vi "List Buckets.vi"() -> ()   [LabVIEW 2015]
doc: "Demonstrates how to list all of the Amazon S3 buckets you own."
uses:
  Typedefs/AMZ_S3_AWS Credentials.ctl
  LV Interface for Amazon S3.lvlib
panel:
  in  "Secret Key":string
  in  "Access Key":string
  out "Buckets":i32(listbox)
  # "Overview: Demonstrates how to list all Amazon S3 buckets created by an authenticated user.\nRequirements: LabVIEW Interface for Amazon S3 toolkit and a registered Amazon AWS account\nInstructions:\n1. Specify the Access Key and Secret Key for your AWS account. You can create an account at http://aws.amazon.com.\n2. Run the VI. All the buckets associated with your account should be listed in the Buckets indicator."
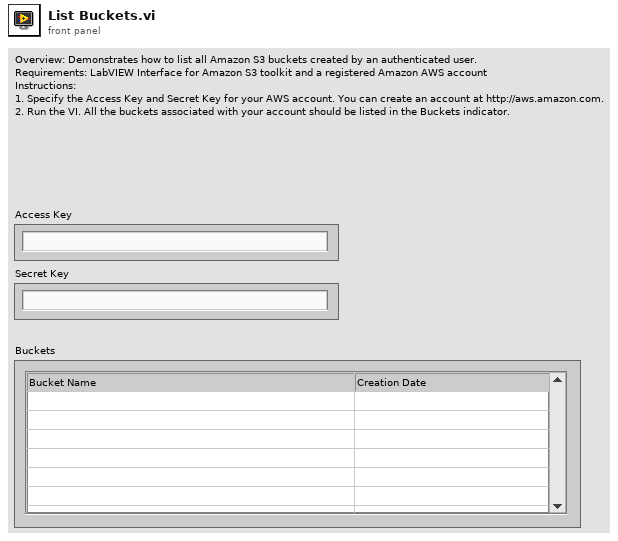
[diagram p1: front panel]
types:
  T1 = typedef "LV Interface for Amazon S3.lvlib/AMZ_S3_AWS Credentials.ctl" = cluster{"Access Key":string, "Secret Key":string}
  T2 = typedef "LV Interface for Amazon S3.lvlib/AMZ_S3_API_Bucket.ctl" = cluster{"Name":string, "CreationDate":timestamp}
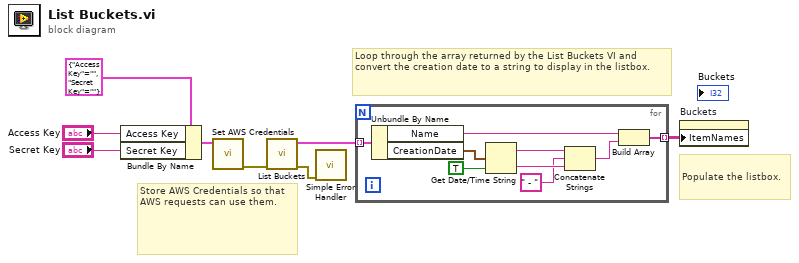
[diagram p0: block diagram]
diagram:
  # "Populate the listbox."
  # "Loop through the array returned by the List Buckets VI and convert the creation date to a string to display in the listbox."
  # "Store AWS Credentials so that AWS requests can use them."
  n1 = Bundle By Name(cluster=T1 {"Access Key"="", "Secret Key"=""} ("AWS Credentials in"), "Access Key"="Access Key", "Secret Key"="Secret Key") -> (w2:T1)
  n2 = call "Set AWS Credentials.vi"("AWS Credentials in"=w2) -> ("error out"=w8:errorcluster)  [unwired: 10 in]
  n3 = call "List Buckets.vi"("error in (no error)"=w8) -> ("error out"=w1:errorcluster, "Buckets"=w7:T2[])  [unwired: 9 in]
  n4 = call <vilib>:"Simple Error Handler.vi"("error in (no error)"=w1) -> ()  [unwired: 4 in, 5 out]
  n5 = for {
    tunnel: w7 -> [w17] mode=indexing
    tunnel: [w9] -> w6 mode=indexing
    n6 = Unbundle By Name(w17) -> ("Name"=w10:string, "CreationDate"=w16:timestamp)
    n7 = Get Date/Time String(seconds (now)=w16, want seconds? (F)=TRUE) -> (date string=w14:string, time string=w13:string)  [unwired: 1 in]
    n8 = Concatenate Strings(w14, " - " ("string"), w13) -> (w11:string)
    n9 = Build Array(w10, w11) -> (w9:string[])
  }
  n10 = property on="Buckets" class="MCListbox (strict)"("ItemNames"=w6) -> ()  [unwired: 2 in, 2 out]
